vi "motor_sim.vi"() -> ()   [LabVIEW 2017]
panel:
  in  "Numeric":dbl
  out "Waveform Chart":dbl(graph)
  in  "stop":bool
  # "Distance 15 0.25 0.06 with 0.2m\nor 7 0.25 0.06 with 5m\nor 2 2 0.06 with 0.5m\nAngle 20 5 0.4 with 0.5 rad"
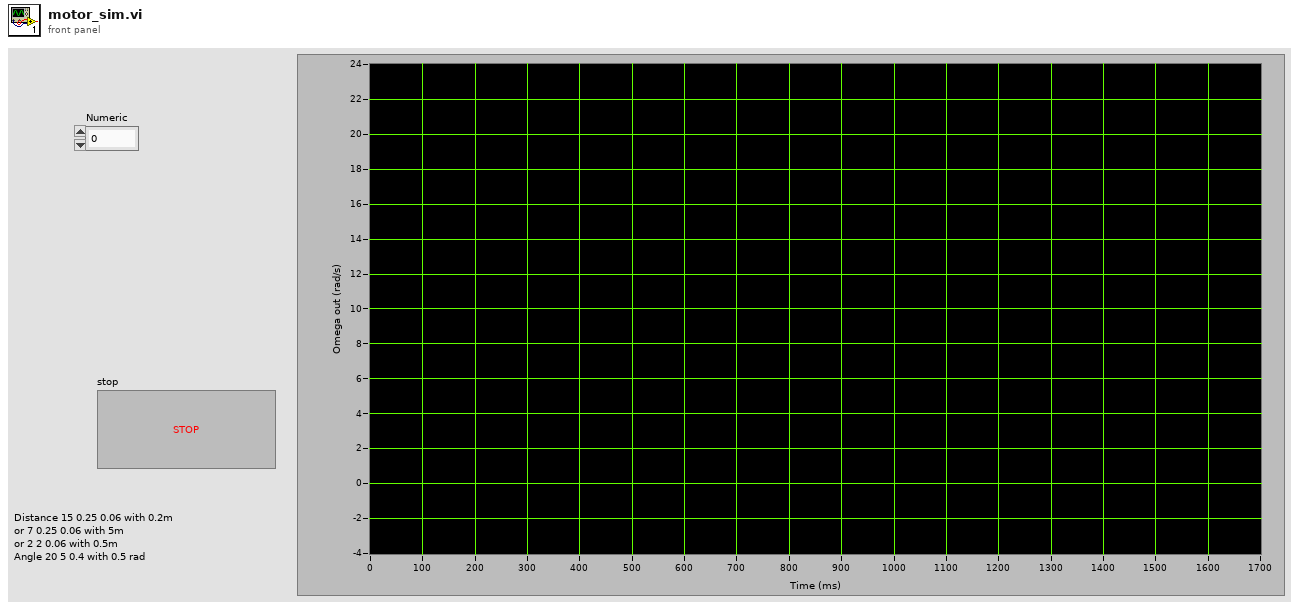
[diagram p1: front panel]
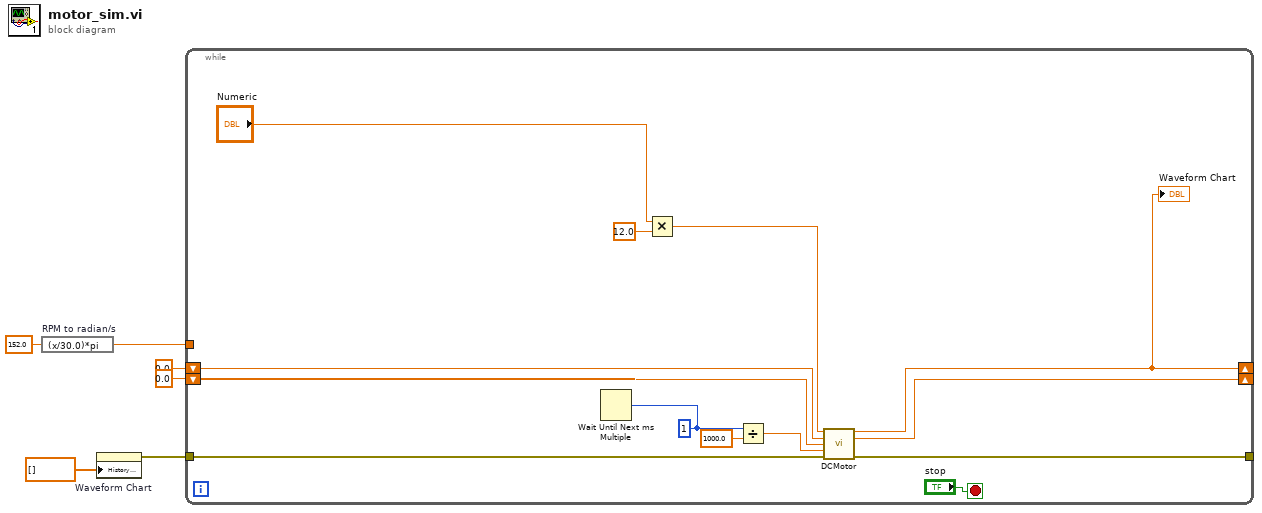
[diagram p0: block diagram]
diagram:
  n1 = expression code="(x/30.0)*pi" "RPM to radian/s"(152.0) -> (w2:dbl)
  n2 = property on="Waveform Chart" class="WFChart (strict)"("History Data"=dbl[] []) -> (error out=w4:errorcluster)  [unwired: 2 in, 1 out]
  n3 = while {
    shift-right: [w9] -> _
    shift-left: 0.0 ("Omega Out") -> [w10]
    shift-right: [w16] -> _
    shift-left: 0.0 ("I Out") -> [w15]
    tunnel: w4 -> [w14]
    tunnel: [w13] -> _
    tunnel: w2 -> [_]
    stop <- "stop" stop-if-true
    w18 = u32 1 ("millisecond multiple")
    n4 = Wait Until Next ms Multiple(millisecond multiple=w18) -> ()  [unwired: 1 out]
    n5 = Multiply(x="Numeric", y=12.0) -> (x*y=w7:dbl)
    n6 = Divide(x=w18, y=1000.0) -> (x/y=w12:dbl)
    n7 = call "DCMotor.vi"("V"=w7, "Omega"=w10, "I"=w15, "dt"=w12, "error in (no error)"=w14) -> ("Omega Out"=w9:dbl, "I Out"=w16:dbl, "error out"=w13:errorcluster)  [unwired: 7 in, 1 out]
    "Waveform Chart" <- w9
  }
